vi "JobDetailMap.Add KeyValue.vi"(8 "error in (no error)":errorcluster, 9 "Value":variant, 10 "Key":string, 11 "Job in":refnum<class "Job.lvclass">) -> (0 "error out":errorcluster, 3 "Job out":refnum<class "Job.lvclass">)   [LabVIEW 2013, in "openCronJob.lvlib" / "Job.lvclass"]
uses:
  Job.lvclass
  Job.lvclass/Job.ctl
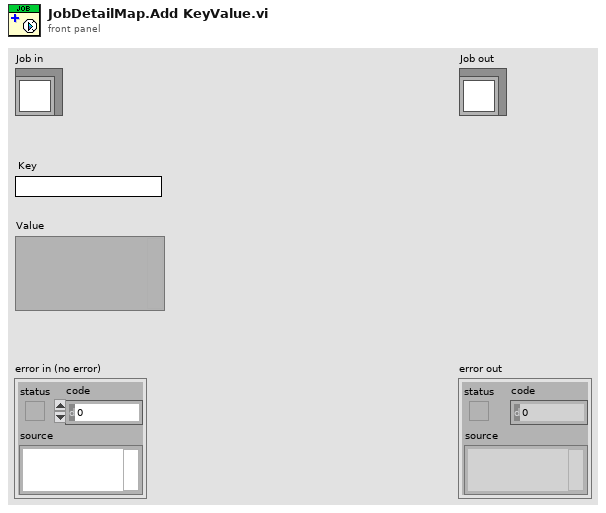
[diagram p1: front panel]
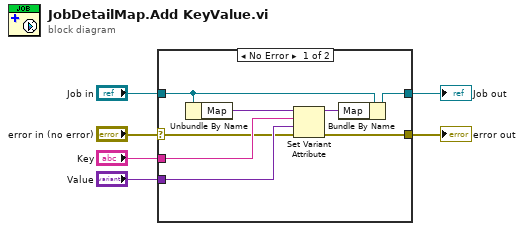
[diagram p0: block diagram]
diagram:
  n1 = case shown="No Error" "error in (no error)" {
    selector: "error in (no error)" -> [w10 w16]
    tunnel: [w9 w16] -> w5
    tunnel: [w8 w15] -> w3
    tunnel: "Job in" -> [w7 w15]
    tunnel: "Key" -> [w13 _]
    tunnel: "Value" -> [w12 _]
    frame No Error {
      n2 = Unbundle By Name(w7) -> ("Map"=w14:variant)
      n3 = Set Variant Attribute(Variant=w14, name=w13, value=w12, error in=w10) -> (Variant out=w11:variant, error out=w9:errorcluster)  [unwired: 1 out]
      n4 = Bundle By Name(cluster=w7, "Map"=w11) -> (w8:refnum<class "Job.lvclass">)
    }
    frame Error {
    }
  }
  "error out" <- w5
  "Job out" <- w3
